vi "Write Value.vi"(8 "error in (no error)":errorcluster, 10 "Value":string, 11 "string in":refnum<class "string.lvclass">) -> (0 "error out":errorcluster, 3 "string out":refnum<class "string.lvclass">)   [LabVIEW 2020, in "Protobuf RAW.lvlib" / "string.lvclass"]
uses:
  string.lvclass
  string.lvclass/string.ctl
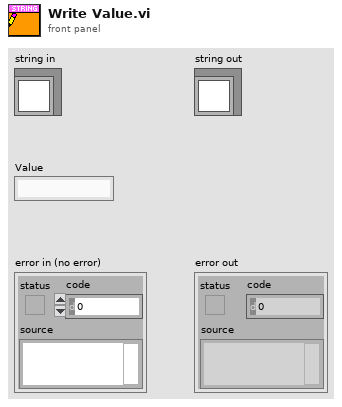
[diagram p1: front panel]
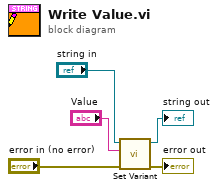
[diagram p0: block diagram]
diagram:
  n1 = call-dynamic "Set Variant.vi"("error in (no error)"="error in (no error)", "Value"="Value", "Proto Type Common in"="string in") -> ("error out"=→"error out":errorcluster, "Proto Type Common out"=→"string out":refnum<class "string.lvclass">)  [unwired: 7 in]
